vi "Write Formatters.vi"(8 "error in (no error)":errorcluster, 10 "Formatters":refnum<class "Formatter Config.lvclass">[](array[class]), 11 "Report Config in":refnum<class "Report Config.lvclass">) -> (0 "error out":errorcluster, 3 "Report Config out":refnum<class "Report Config.lvclass">)   [LabVIEW 2015, in "Report Config.lvclass"]
uses:
  Report Config.lvclass
  Report Formatters/Base Class/Config/Formatter Config.lvclass
  Report Config.lvclass/Report Config.ctl
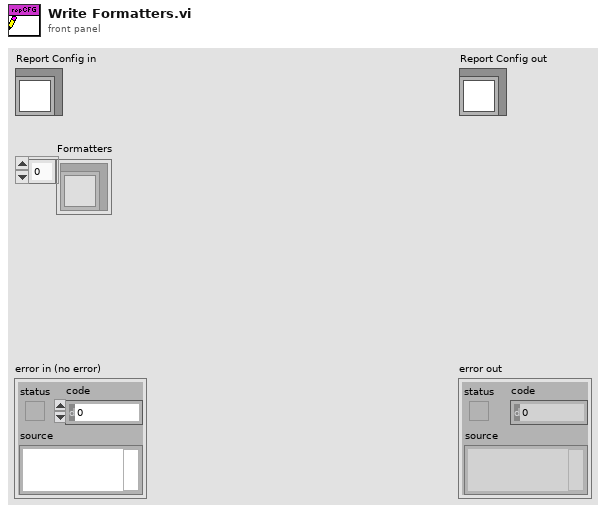
[diagram p1: front panel]
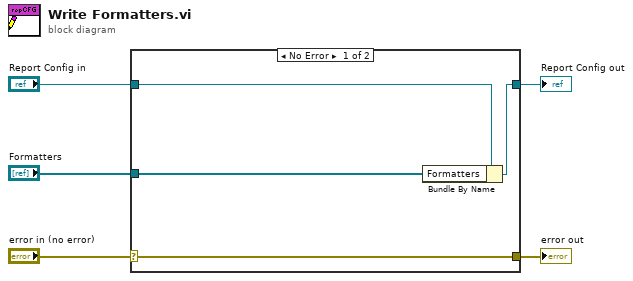
[diagram p0: block diagram]
diagram:
  n1 = case shown="No Error" "error in (no error)" {
    selector: "error in (no error)" -> [w9 w10]
    tunnel: [w9 w10] -> w4
    tunnel: [w7 w11] -> w2
    tunnel: "Report Config in" -> [w8 w11]
    tunnel: "Formatters" -> [w6 _]
    frame No Error {
      n2 = Bundle By Name(cluster=w8, "Formatters"=w6) -> (w7:refnum<class "Report Config.lvclass">)
    }
    frame Error {
    }
  }
  "error out" <- w4
  "Report Config out" <- w2
